vi "test_TwoSessTwoPinTwoInstrTwoSiteReservation_CallNiFgenGetConnections1Pin1Connection_ReturnsOneConnection.vi"(8 "error in":errorcluster) -> (0 "error out":errorcluster, 2 "result":string, 3 "pass":bool)   [LabVIEW 2020, in "MeasurementServerTests.lvlib"]
uses:
  MeasurementServerTests.lvlib
  Runtime/APIs/Session Management V1/Session Reservation/Connection.ctl
  Runtime/APIs/Session Management V1/Session Reservation/Session Reservation.lvclass
  03fc85e1-696b-4ece-a78b-f41470766ac0.vi
  Runtime/Sessions/niFGEN Sessions/Plug-In SDK niFGEN Sessions.lvlib
  Runtime/Sessions/niFGEN Sessions/Get Connections - 1Pin 1Conn.vi
  Runtime/Sessions/niFGEN Sessions/Connection with Session.ctl
  ee969218-a503-4951-836c-6bb19e4d29f5.vi
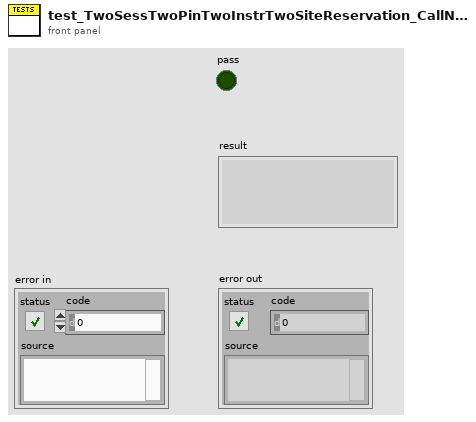
[diagram p1: front panel]
types:
  T1 = typedef "Plug-In SDK niFGEN Sessions.lvlib/Connection with Session.ctl" = cluster{"connection":T2, "session":refnum<k15>}
  T2 = typedef "Plug-In SDK Session Management V1 API.lvlib/Session Reservation.lvclass/Connection.ctl" = cluster{"pin or relay name":string, "site":i32, "instrument type id":string, "channel":string}
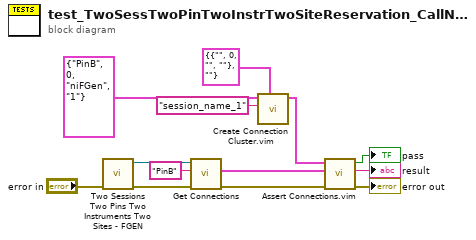
[diagram p0: block diagram]
diagram:
  n1 = call "Two Sessions Two Pins Two Instruments Two Sites - FGEN.vi"("error in"="error in") -> ("error out"=w5:errorcluster, "session reservation out"=w6:refnum<class "Session Reservation.lvclass">)  [unwired: 9 in]
  n2 = call-poly "Get Connections.vi"("error in"=w5, "pin or relay name"="PinB", "session reservation in"=w6) -> ("error out"=w4:errorcluster, "connection"=w1:T1)  [unwired: 6 in, 1 out]
  n3 = call "Create Connection Cluster.vim"("connection type"=T1 {"connection"={"pin or relay name"="", "site"=0, "instrument type id"="", "channel"=""}, "session"=""} ("niDCPower connection"), "session in"="session_name_1", "hardware independent connection in"=T2 {"pin or relay name"="PinB", "site"=0, "instrument type id"="niFGen", "channel"="1"} ("connection")) -> ("connection out"=w2:T1)  [unwired: 8 in]
  n4 = call "Assert Connections.vim"("error in"=w4, "actual connections"=w1, "expected connections"=w2) -> ("error out"=→"error out":errorcluster, "result"=→"result":string, "pass"=→"pass":bool)  [unwired: 6 in]
